vi "Write OpenFPWhenCreated Key.vi"(8 "Error In":errorcluster, 11 "\"Open FP When Created?\" ticked by default?":enum32{"Yes", "No"}(ring)) -> (0 "Error Out":errorcluster)   [LabVIEW 2022 SP3]
doc: "This VI creates the \"HKEY_CURRENT_USER\\Software\\NewViFromTemplate_LabVIEW_IDE_Extension\" subkey, and writes the \"OpenFrontPanelWhenNewViCreated\" value."
uses:
  <vilib>/registry/registry.llb/Write Registry Value Simple STR.vi
panel:
  # "Development\nControls or indicators that are useful for development or testing, but which are not outputs of the VI."
  # "Input\nInputs to the VI"
  # "Output\nOutputs of the VI"
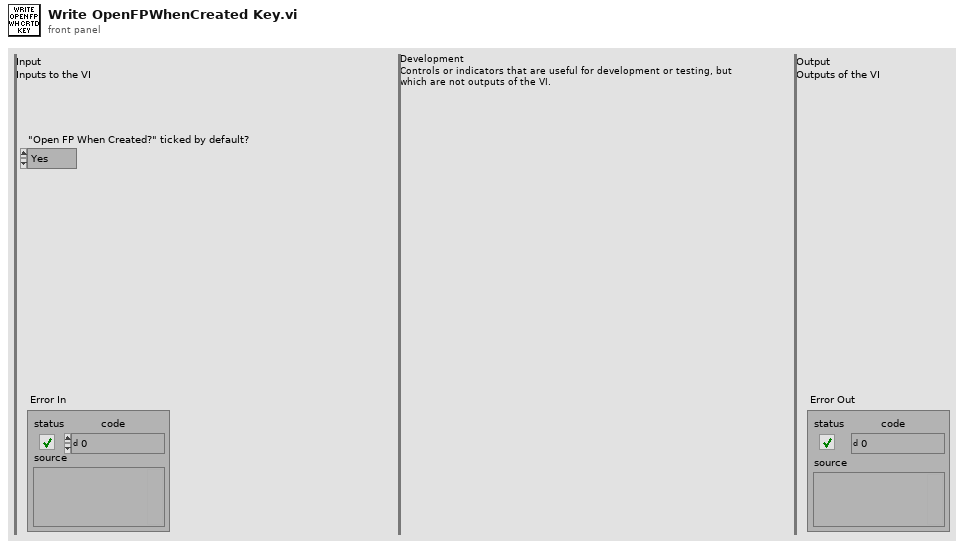
[diagram p1: front panel]
types:
  T1 = typedef "Registry RtKey.ctl" = enum32{"HKEY_CLASSES_ROOT", "HKEY_CURRENT_USER", "HKEY_LOCAL_MACHINE", "HKEY_USERS", "HKEY_PERFORMANCE_DATA", "HKEY_CURRENT_CONFIG", "HKEY_DYN_DATA"}
  T2 = typedef "Registry refnum.ctl" = refnum<k1>
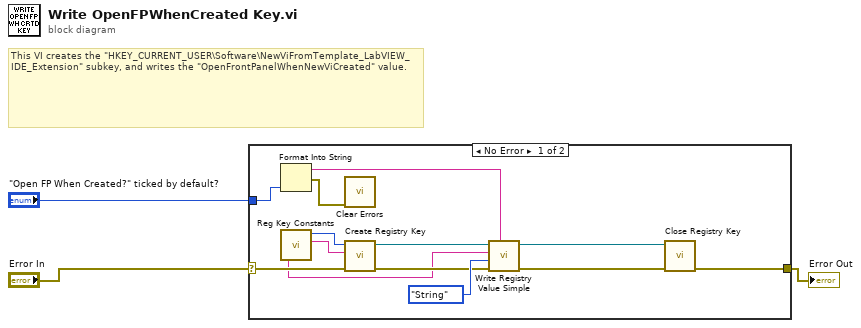
[diagram p0: block diagram]
diagram:
  # "This VI creates the \"HKEY_CURRENT_USER\\Software\\NewViFromTemplate_LabVIEW_IDE_Extension\" subkey, and writes the \"OpenFrontPanelWhenNewViCreated\" value."
  n1 = case shown="No Error" "Error In" {
    selector: "Error In" -> [w11 w17]
    tunnel: [w8 w17] -> w2
    tunnel: "\"Open FP When Created?\" ticked by default?" -> [w6 _]
    frame No Error {
      n2 = Format Into String(w6) -> (resulting string=w4:string, error out=w5:errorcluster)  [unwired: 3 in]
      n3 = call "Reg Key Constants.vi"() -> ("Subkey Path"=w16:string, "Root Key"=w15:T1, "Name of OpenFrontPanelWhenNewViCreated Value"=w7:string)  [unwired: 3 in, 2 out]
      n4 = call <vilib>:"Clear Errors.vi"("error in (no error)"=w5) -> ()  [unwired: 5 in, 2 out]
      n5 = call <vilib>:"Create Registry Key.vi"("error in (no error)"=w11, "subkey"=w16, "root key (HKEY_LOCAL_MACHINE)"=w15) -> ("error out"=w10:errorcluster, "refnum out"=w14:T2)  [unwired: 6 in, 1 out]
      n6 = call-poly <vilib>:"Write Registry Value Simple.vi"("String/Binary data"=w4, "error in (no error)"=w10, "simple data type"=enum16{"String", "Binary", "DWORD"}."String", "value"=w7, "refnum"=w14) -> ("error out"=w9:errorcluster, "refnum out"=w13:T2)  [unwired: 3 in]
      n7 = call <vilib>:"Close Registry Key.vi"("error in (no error)"=w9, "refnum"=w13) -> ("error out"=w8:errorcluster)  [unwired: 5 in]
    }
    frame Error {
    }
  }
  "Error Out" <- w2
